vi "Boiler_Startup_Control.vi"() -> ()   [LabVIEW 2021]
doc: "This is the Main Vi that performs the boiler startup operation."
uses:
  Controls/Queue_Operation_Select.ctl
  Controls/Timer_Operation_Select.ctl
  Controls/State_and_Data.ctl
  Controls/Boiler_Status_Indicators.ctl
  Controls/Notifier_Operation_Select.ctl
  Controls/Boiler_Data.ctl
  <vilib>/Utility/file.llb/Write Delimited Spreadsheet (string).vi
panel:
  out "Boiler_Status_Indicators":T1 caption="Boiler Status Indicators"
  in  "Stop":bool
  in  "Forced_Draft_Fan":bool caption="Forced Draft Fan"
  in  "Run_Interlock":bool caption="Run Interlock"
  in  "Flame_Sensor_Value":dbl(slide) caption="Flame Sensor Value [%]" scale=0.0..100.0
  in  "Fuel_Control_Valve":dbl(knob) caption="Fuel  Control Valve Position [% Open]" scale=0.0..100.0 scale format="%.1f"
  in  "Shutdown":bool
  in  "Pilot":bool
  in  "Start_Sequence":bool caption="Start Sequence"
  in  "Boiler_Reset":bool caption="Boiler Reset"
  out "Error_Out":errorcluster
  in  "Error_In":errorcluster
  # "Boiler Controls"
  # "Boiler Simulation Controls"
  # "Closed"
  # "On"
  # "Open"
  # "Off"
  # "Boiler Start-Up steps\nStep1 : Close the interlock and hit the reset button.\nStep2 : Press the start sequence to initiate the pre-purge. \nStep3 : After the pre-purge, press the pilot button to turn on the natural gas and pilot.\nStep4 : Adjust the flame sensor to prepare the boiler.\nStep5 : Turn on the forced draft fan, then add fuel to the boiler by adjusting the fuel control valve.\nStep6 :The boiler is now started up"
  # "Seconds"
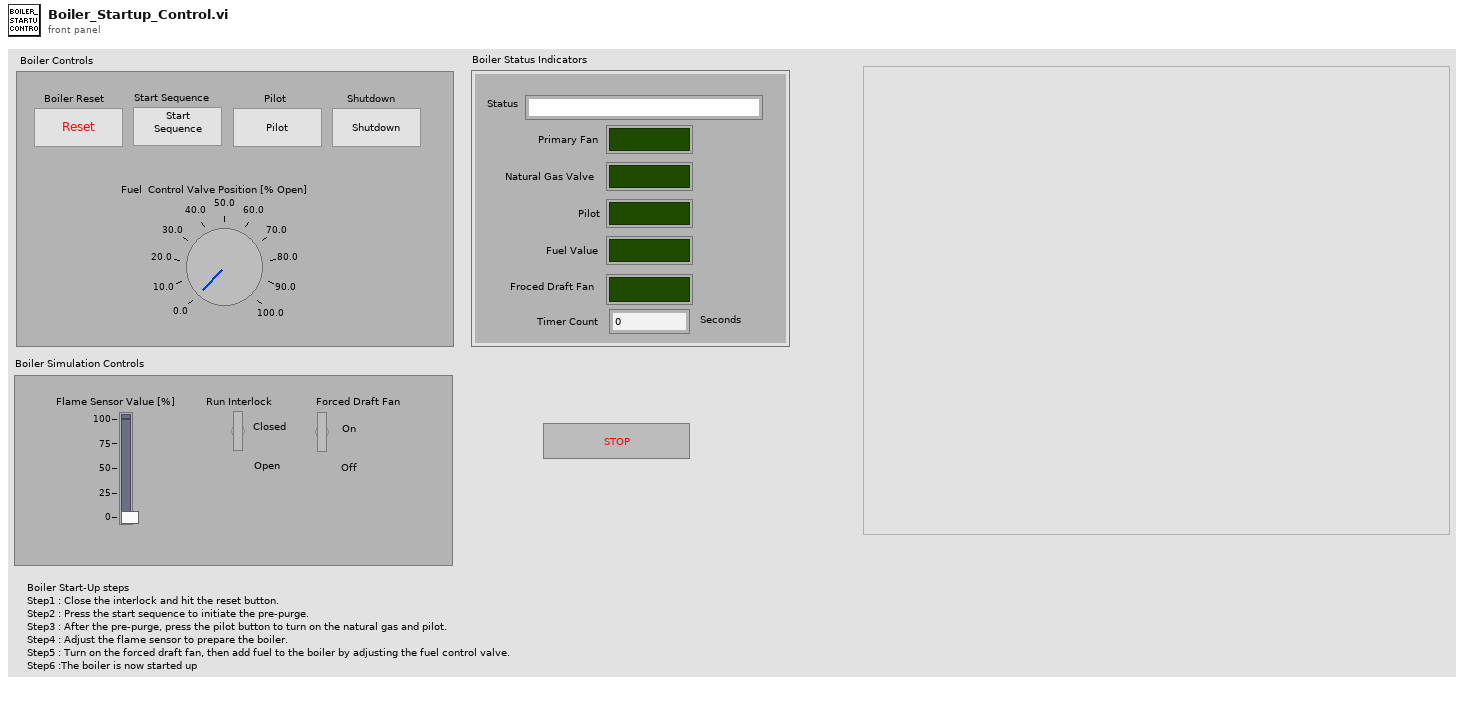
[diagram p1: front panel]
types:
  T1 = typedef "Boiler_Status_Indicators.ctl" = cluster{"Status":string, "Primary_Fan":bool, "Natural_Gas_Valve":bool, "Pilot":bool, "Fuel_Value":bool, "Froced_Draft_Fan":bool, "Timer_Count":dbl}
  T2 = typedef "Notifier_Operation_Select.ctl" = enum16{"Obtain_Notifier", "Send_Notification", "Get_Notification_Status", "Release_Notifier"}
  T3 = typedef "Queue_Operation_Select.ctl" = enum16{"Obtain_Queue", "Enqueue", "Enqueue_N", "Enqueue_at_First", "Dequeue", "Flush_Queue", "Release_Queue"}
  T4 = typedef "State_and_Data.ctl" = cluster{"State":string, "Event_Data":variant}
  T5 = typedef "Boiler_Data.ctl" = cluster{"Boiler_Status_Indicators":T1, "Start?":bool, "Pilot_On?":bool, "Blink_It?":bool, "Log_Timer_Time":bool, "ReInitialize":refnum<vi>[], "After_TimeOut_Call?":string, "Time_String":string, "Event_String":string, "Event_Data_String":string}
  T6 = typedef "Timer_Operation_Select.ctl" = enum16{"Start_Timer", "Pause_Timer", "Time_Out?", "Stop_Timer"}
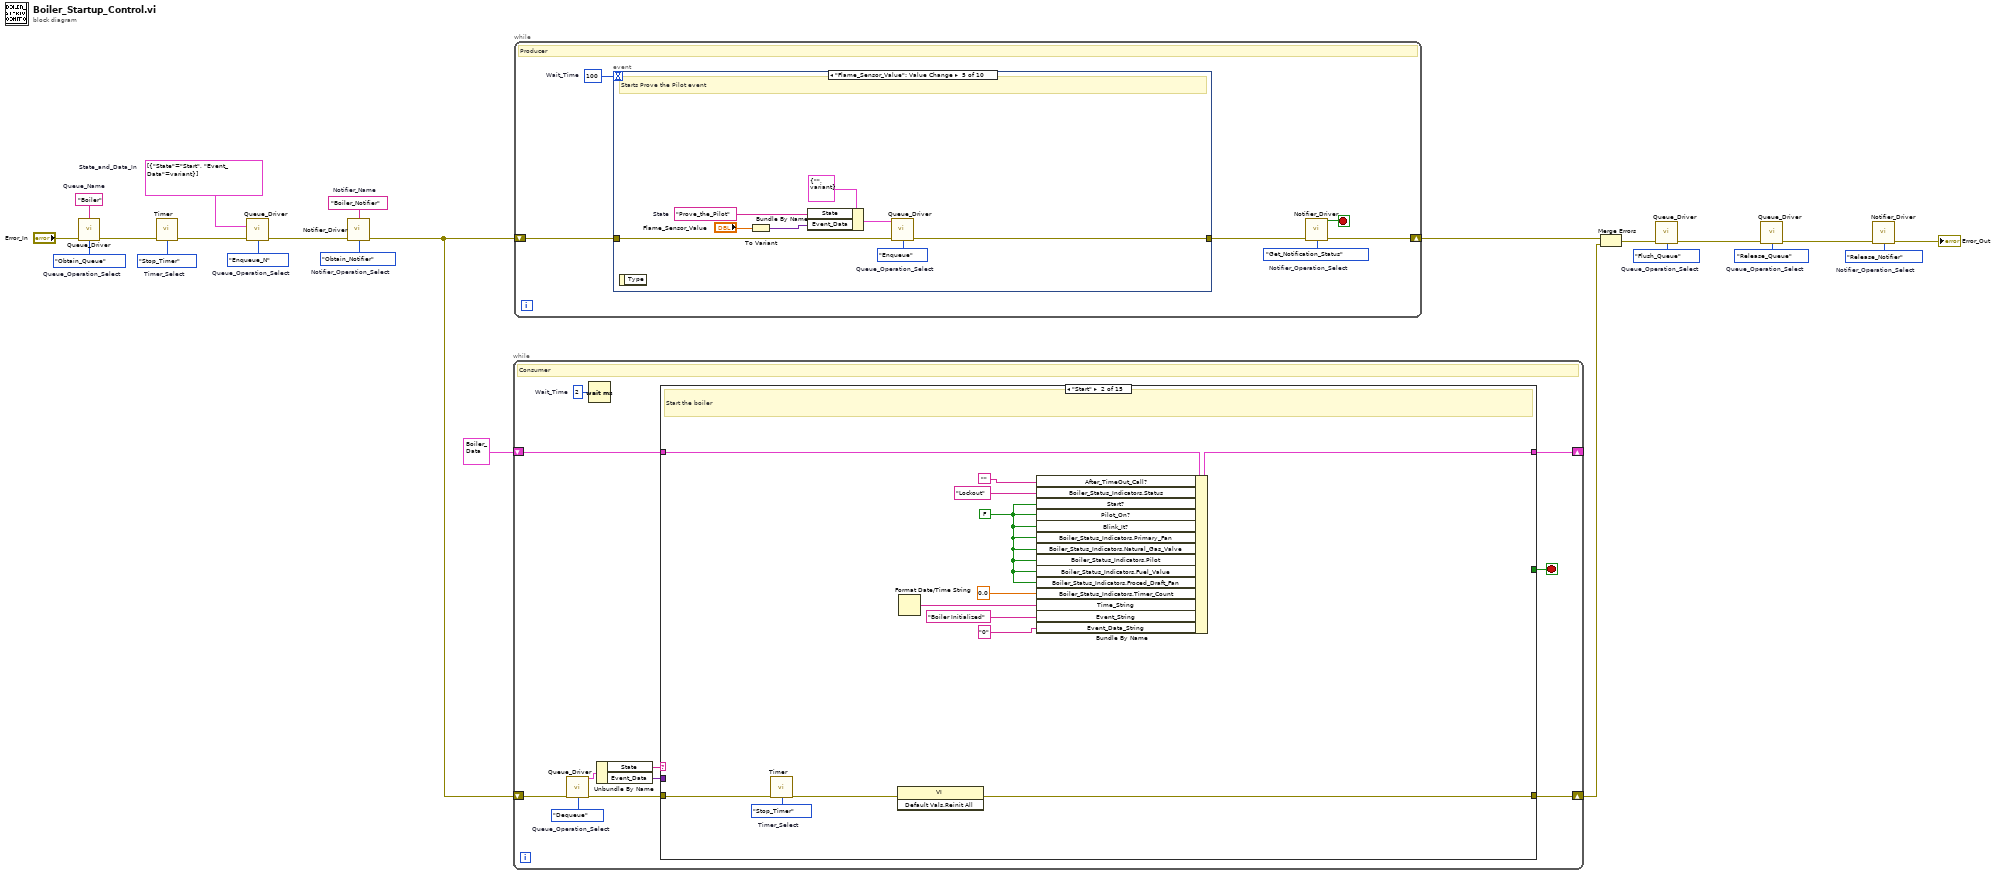
[diagram p0: block diagram]
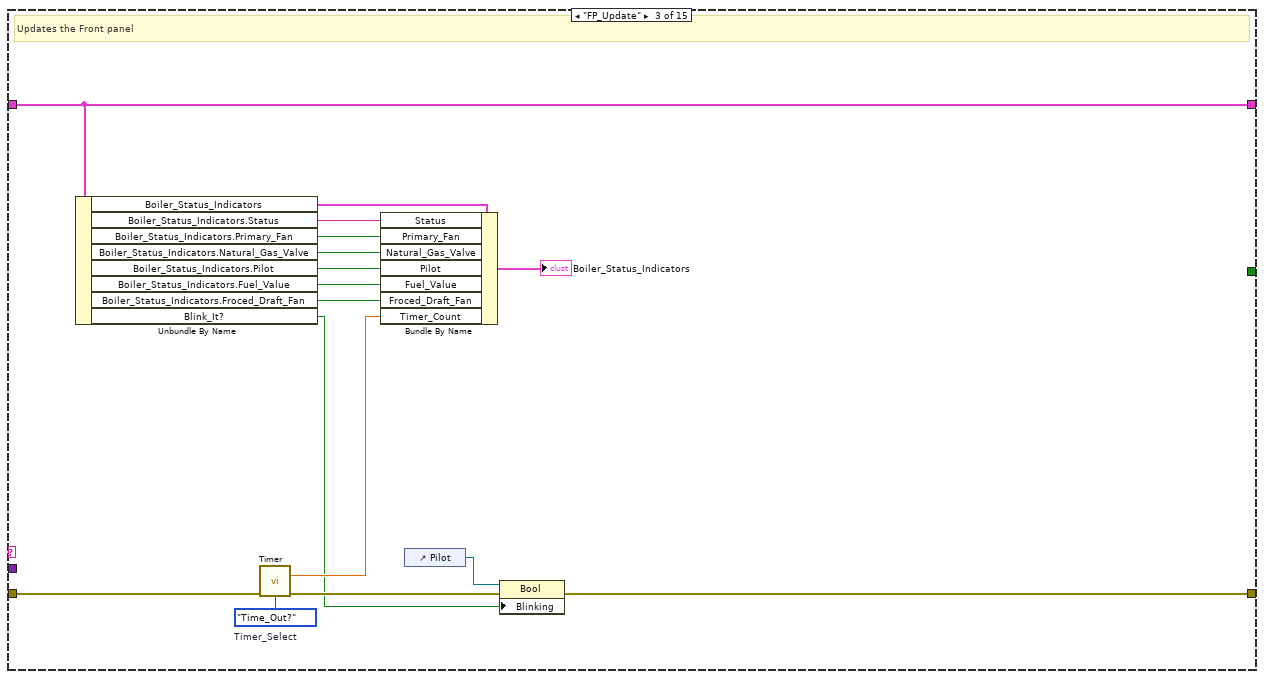
[diagram p3: hidden frame]
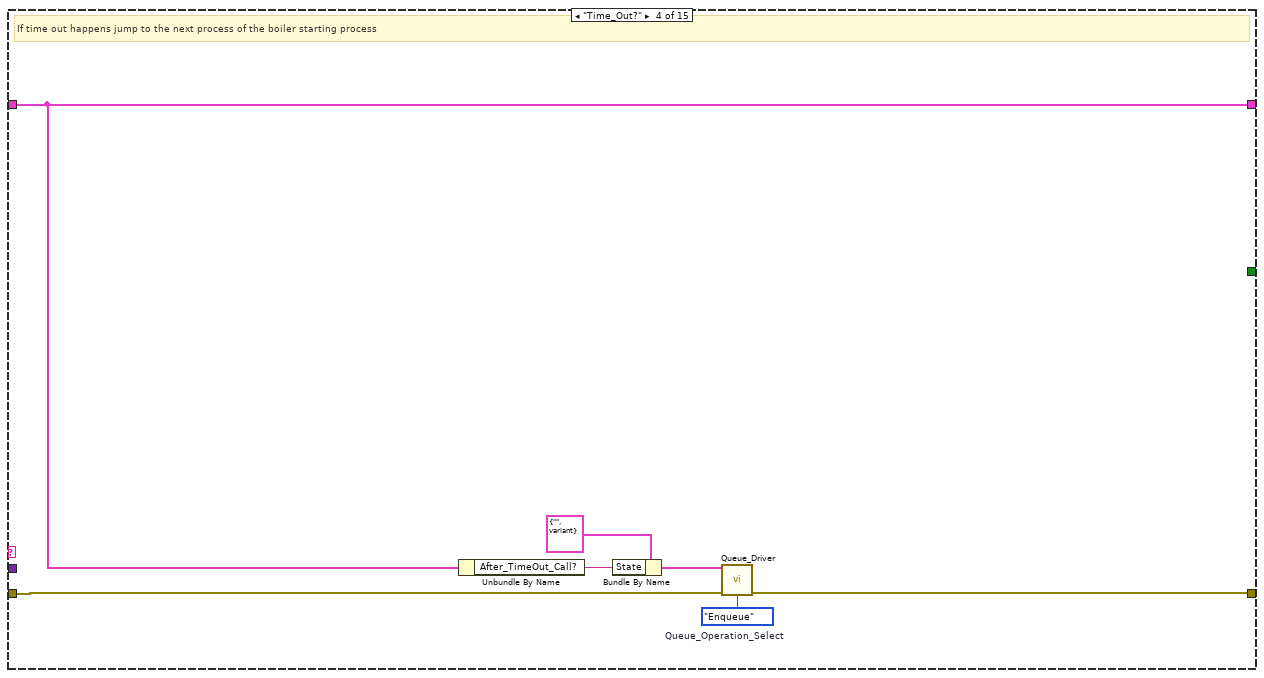
[diagram p4: hidden frame]
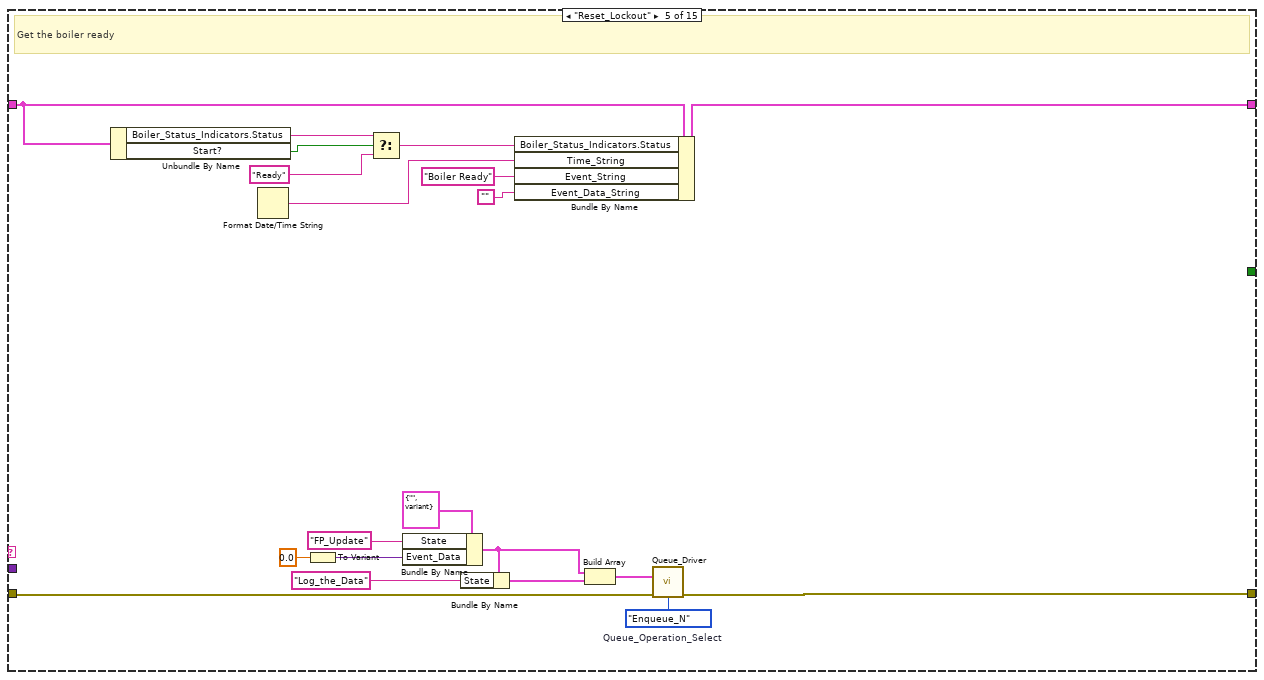
[diagram p5: hidden frame]
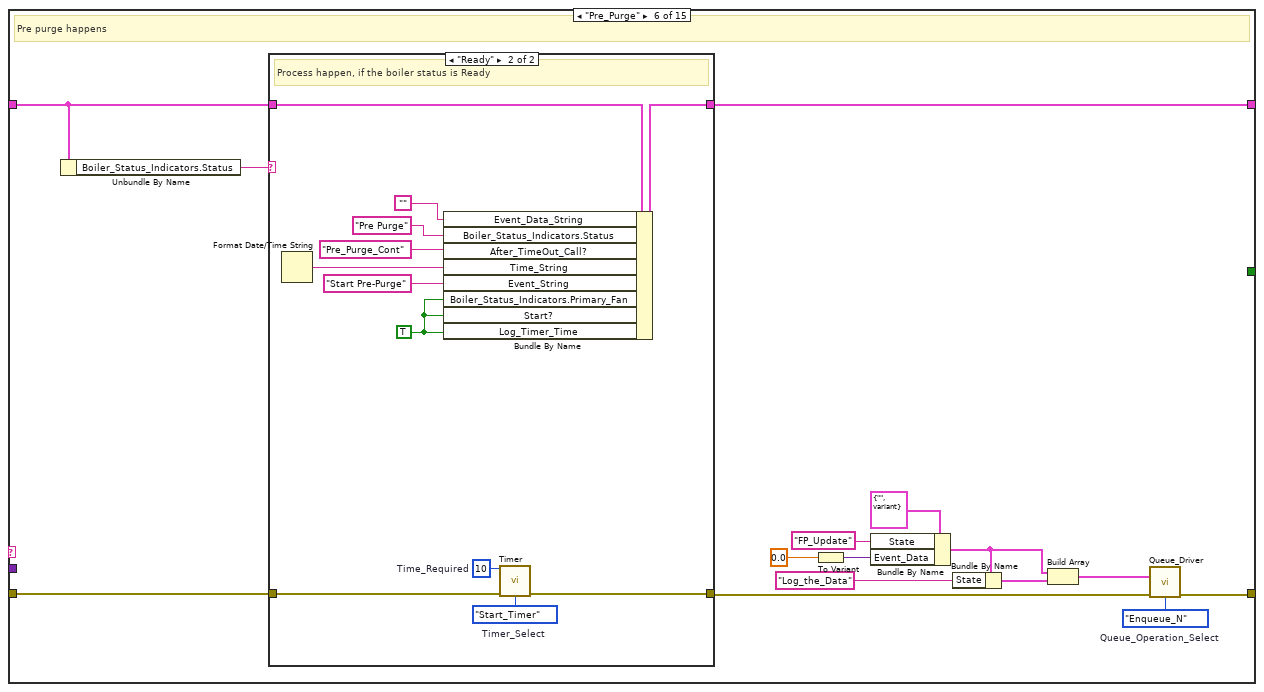
[diagram p6: hidden frame]
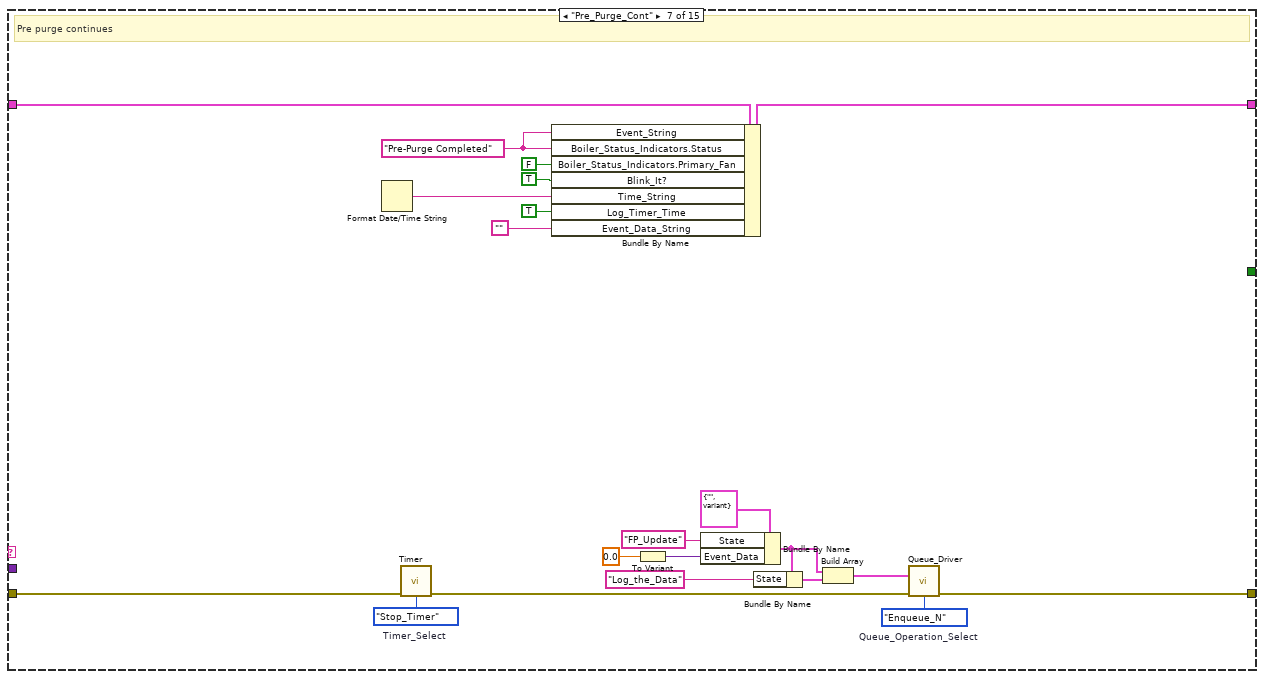
[diagram p8: hidden frame]
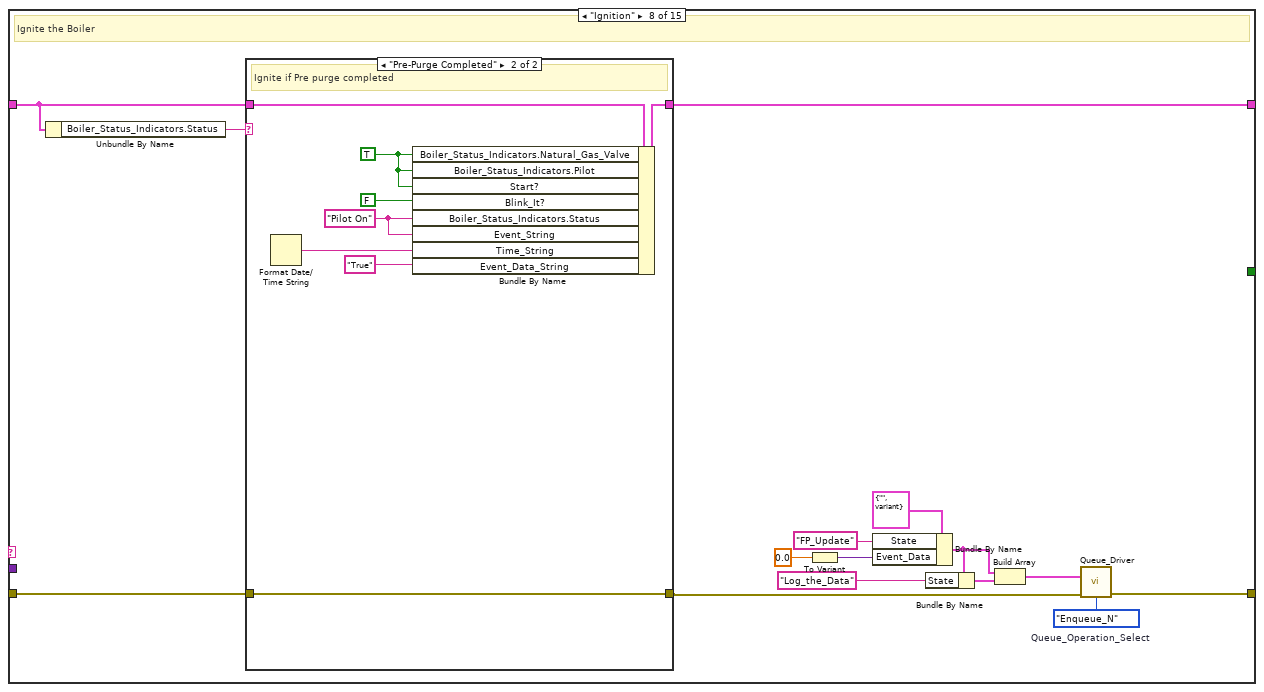
[diagram p9: hidden frame]
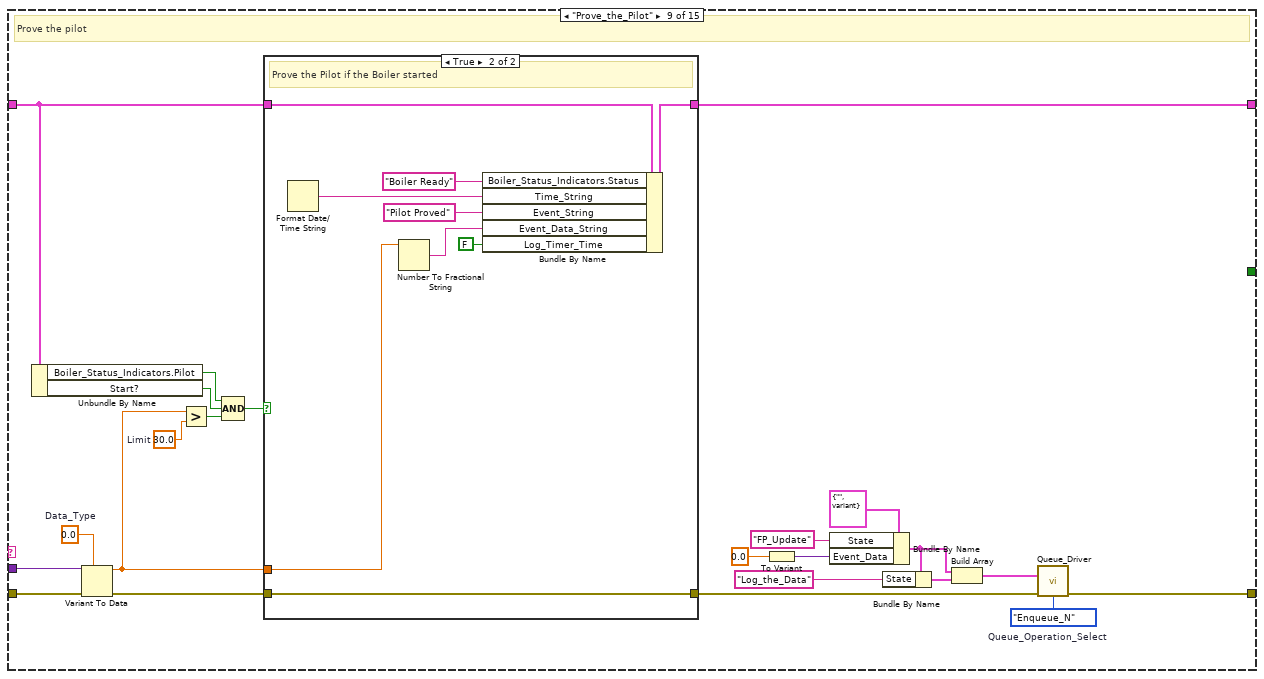
[diagram p11: hidden frame]
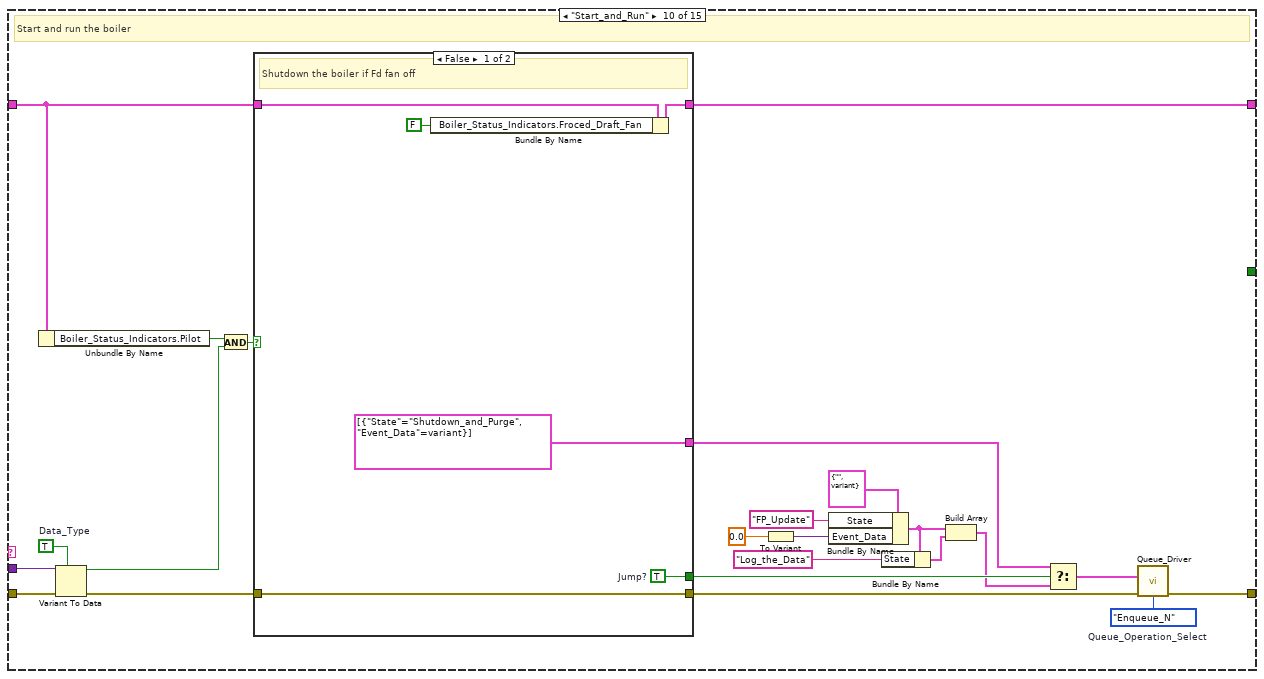
[diagram p13: hidden frame]
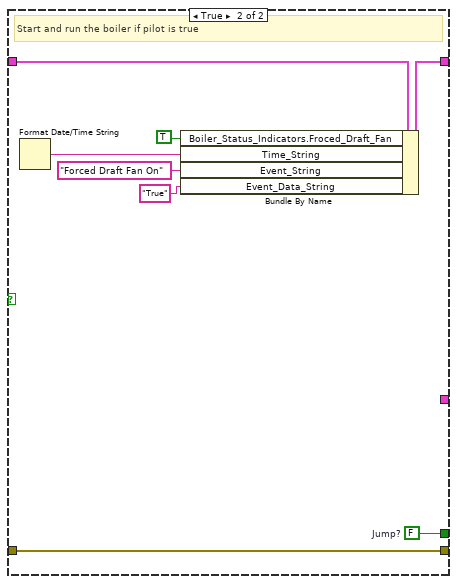
[diagram p14: hidden frame]
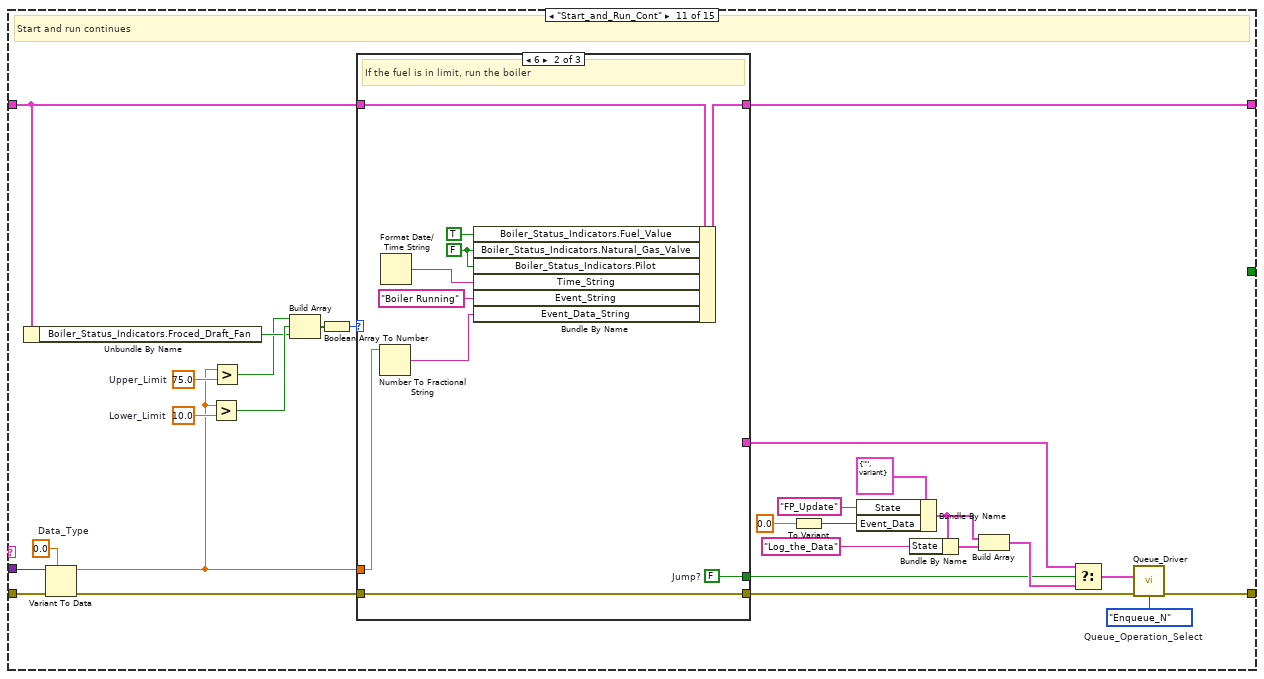
[diagram p15: hidden frame]
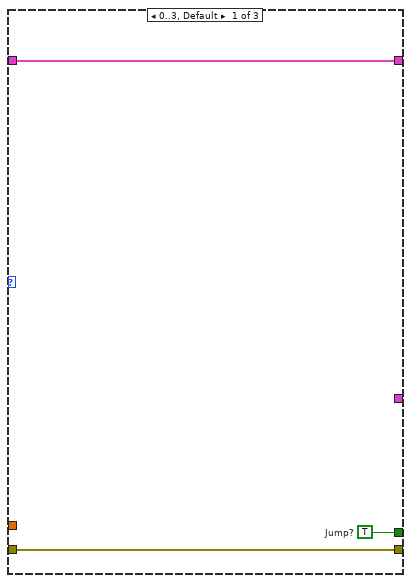
[diagram p16: hidden frame]
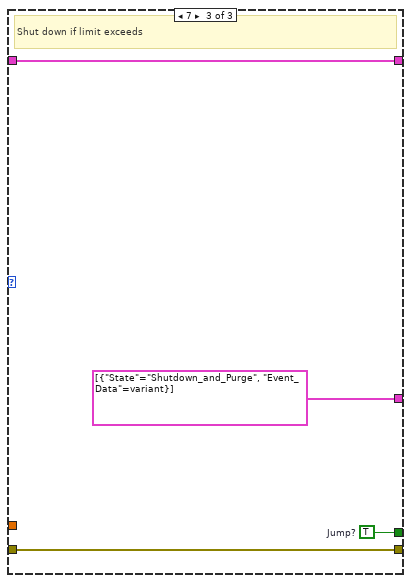
[diagram p17: hidden frame]
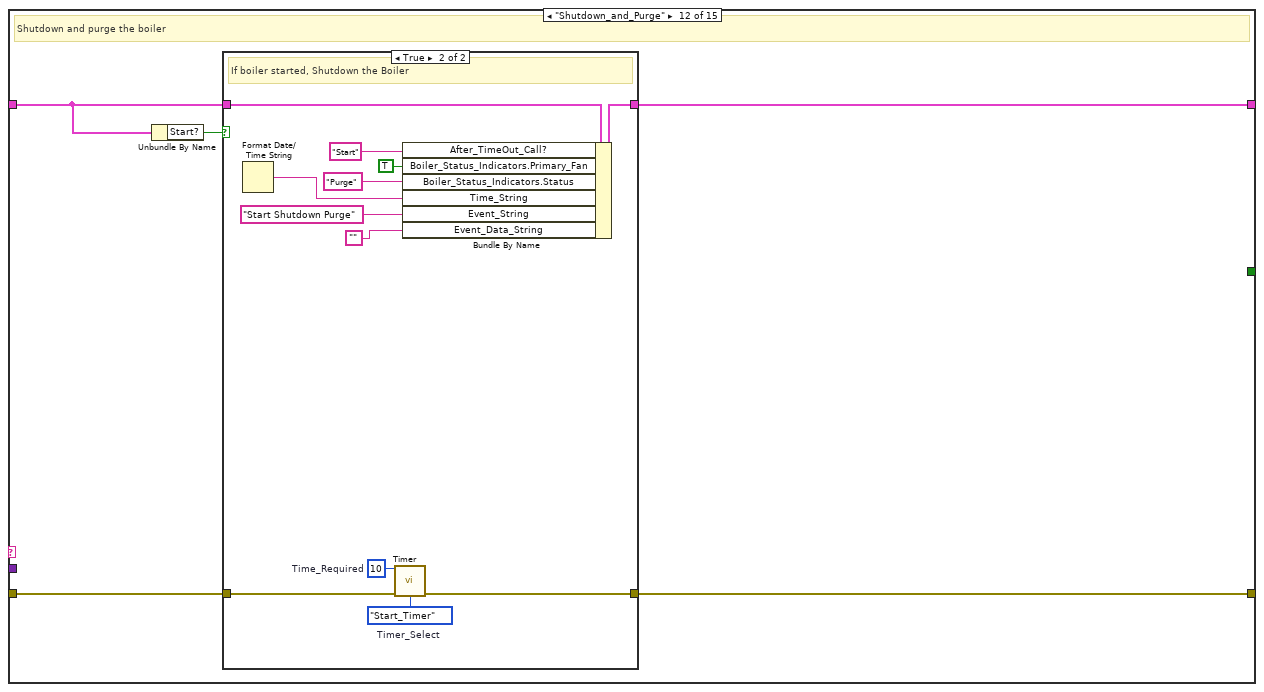
[diagram p18: hidden frame]
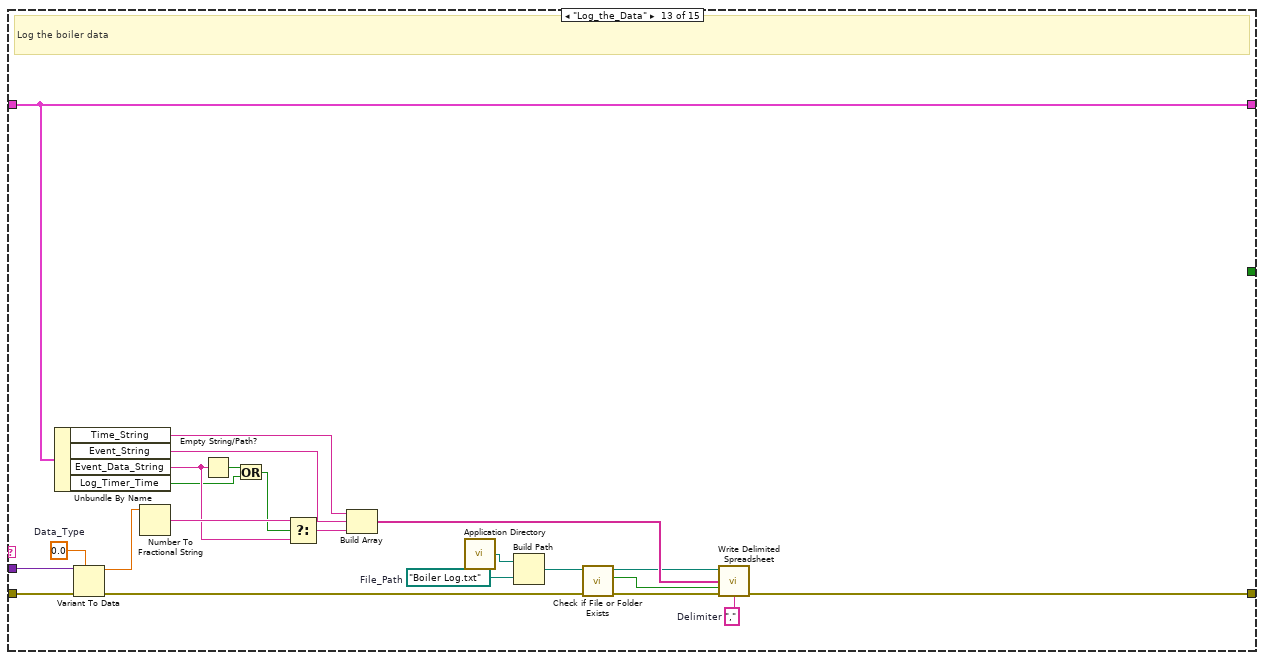
[diagram p20: hidden frame]
diagram:
  w5 = Notifier_Operation_Select."Release_Notifier"  # Notifier_Operation_Select
  w6 = Queue_Operation_Select."Release_Queue"  # Queue_Operation_Select
  w8 = Queue_Operation_Select."Flush_Queue"  # Queue_Operation_Select
  w10 = "Boiler_Notifier"  # Notifier_Name
  w11 = Notifier_Operation_Select."Obtain_Notifier"  # Notifier_Operation_Select
  w13 = T4[] [{"State"="Start", "Event_Data"=variant}]  # State_and_Data_In
  w14 = Queue_Operation_Select."Enqueue_N"  # Queue_Operation_Select
  w18 = Timer_Operation_Select."Stop_Timer"  # Timer_Select
  w19 = "Boiler"  # Queue_Name
  w20 = Queue_Operation_Select."Obtain_Queue"  # Queue_Operation_Select
  n1 = call "Queue_Driver.vi"("Queue_Name"=w19, "Error_In"="Error_In", "Queue_Operation_Select"=w20) -> ("Error_Out"=w21:errorcluster)  [unwired: 11 in, 1 out]
  n2 = call "Timer.vi"("Error_In"=w21, "Timer_Select"=w18) -> ("Error_Out"=w17:errorcluster)  [unwired: 10 in, 3 out]
  n3 = call "Queue_Driver.vi"("State_and_Data_In_N"=w13, "Error_In"=w17, "Queue_Operation_Select"=w14) -> ("Error_Out"=w15:errorcluster)  [unwired: 11 in, 1 out]
  n4 = call "Notifier_Driver.vi"("Notifier_Name"=w10, "Error_In"=w15, "Notifier_Operation_Select"=w11) -> ("Error_Out"=w12:errorcluster)  [unwired: 11 in, 1 out]
  n5 = while {
    shift-right: [w28] -> _
    shift-left: T5 {"Boiler_Status_Indicators"={"Status"="", "Primary_Fan"=FALSE, "Natural_Gas_Valve"=FALSE, "Pilot"=FALSE, "Fuel_Value"=FALSE, "Froced_Draft_Fan"=FALSE, "Timer_Count"=0.0}, "Start?"=TRUE, "Pilot_On?"=TRUE, "Blink_It?"=TRUE, "Log_Timer_Time"=FALSE, "ReInitialize"=[], "After_TimeOut_Call?"="", "Time_String"="", "Event_String"="", "Event_Data_String"=""} -> [w27]
    shift-right: [w23] -> w4
    shift-left: w12 -> [w33]
    stop <- w25 stop-if-true
    w24 = u32 2  # Wait_Time
    w31 = Queue_Operation_Select."Dequeue"  # Queue_Operation_Select
    # "Consumer"
    n6 = call "Queue_Driver.vi"("Error_In"=w33, "Queue_Operation_Select"=w31) -> ("State_and_Data_Out"=w30:T4, "Error_Out"=w32:errorcluster)  [unwired: 12 in]
    n7 = Wait (ms)(milliseconds to wait=w24) -> ()  [unwired: 1 out]
    n8 = Unbundle By Name(w30) -> ("State"=w29:string, "Event_Data"=w26:variant)
    n9 = case shown="\"Start\"" w29 {
      tunnel: w32 -> [w35 w41 w64 w68 w74 w105 w137 w154 w188 w222 w262 w286 w319 w331 w340]
      tunnel: [w35 w40 w49 w67 w73 w94 w136 w141 w167 w204 w240 w284 w323 w329 w335] -> w23
      tunnel: [w34 w48 w63 w70 w91 w106 w140 w155 w179 w221 w264 w285 w320 w330 w351] -> w28
      tunnel: w27 -> [w34 w47 w63 w70 w89 w104 w138 w153 w180 w220 w263 w283 w320 w330 w351]
      tunnel: w26 -> [_ _ _ _ _ _ _ _ w187 w217 w260 _ w318 _ _]
      tunnel: [_ _ _ _ _ _ _ _ _ _ _ _ _ w324 _] -> w25
      frame Default {
        # "Default"
      }
      frame "Start" {
        w37 = Timer_Operation_Select."Stop_Timer"  # Timer_Select
        w42 = FALSE ("Boiler_Status_Indicators.Primary_Fan")
        # "Start the boiler"
        n10 = call "Timer.vi"("Error_In"=w41, "Timer_Select"=w37) -> ("Error_Out"=w38:errorcluster)  [unwired: 10 in, 3 out]
        n11 = invoke on="Invoke Node" class="VI" method="Default Vals.Reinit All"(error in=w38) -> (error out=w40:errorcluster)  [unwired: 2 in, 2 out]
        n12 = Format Date/Time String() -> (date/time string=w36:string)  [unwired: 3 in]
        n13 = Bundle By Name(cluster=w47, "After_TimeOut_Call?"="" ("Empty String Constant"), "Boiler_Status_Indicators.Status"="Lockout", "Start?"=w42, "Pilot_On?"=w42, "Blink_It?"=w42, "Boiler_Status_Indicators.Primary_Fan"=w42, "Boiler_Status_Indicators.Natural_Gas_Valve"=w42, "Boiler_Status_Indicators.Pilot"=w42, "Boiler_Status_Indicators.Fuel_Value"=w42, "Boiler_Status_Indicators.Froced_Draft_Fan"=w42, "Boiler_Status_Indicators.Timer_Count"=0.0, "Time_String"=w36, "Event_String"="Boiler Initialized", "Event_Data_String"="0") -> (w48:T5)
      }
      frame "FP_Update" {
        w54 = Timer_Operation_Select."Time_Out?"  # Timer_Select
        # "Updates the Front panel"
        n14 = Unbundle By Name(w63) -> ("Boiler_Status_Indicators"=w62:T1, "Boiler_Status_Indicators.Status"=w61:string, "Boiler_Status_Indicators.Primary_Fan"=w60:bool, "Boiler_Status_Indicators.Natural_Gas_Valve"=w59:bool, "Boiler_Status_Indicators.Pilot"=w58:bool, "Boiler_Status_Indicators.Fuel_Value"=w57:bool, "Boiler_Status_Indicators.Froced_Draft_Fan"=w56:bool, "Blink_It?"=w51:bool)
        n15 = call "Timer.vi"("Error_In"=w64, "Timer_Select"=w54) -> ("Time"=w52:dbl, "Error_Out"=w55:errorcluster)  [unwired: 10 in, 2 out]
        n16 = Bundle By Name(cluster=w62, "Status"=w61, "Primary_Fan"=w60, "Natural_Gas_Valve"=w59, "Pilot"=w58, "Fuel_Value"=w57, "Froced_Draft_Fan"=w56, "Timer_Count"=w52) -> (→"Boiler_Status_Indicators":T1)
        n17 = control-ref of="Pilot"() -> (w50:refnum<vi>)
        n18 = property on="Property Node" class="Bool"(reference=w50, error in=w55, "Blinking"=w51) -> (error out=w49:errorcluster)  [unwired: 1 out]
      }
      frame "Time_Out?" {
        w66 = Queue_Operation_Select."Enqueue"  # Queue_Operation_Select
        # "If time out happens jump to the next process of the boiler starting process"
        n19 = Unbundle By Name(w70) -> ("After_TimeOut_Call?"=w71:string)
        n20 = Bundle By Name(cluster=T4 {"State"="", "Event_Data"=variant} ("State_and_Data_In"), "State"=w71) -> (w65:T4)
        n21 = call "Queue_Driver.vi"("State_and_Data_In"=w65, "Error_In"=w68, "Queue_Operation_Select"=w66) -> ("Error_Out"=w67:errorcluster)  [unwired: 11 in, 1 out]
      }
      frame "Reset_Lockout" {
        w82 = Queue_Operation_Select."Enqueue_N"  # Queue_Operation_Select
        # "Get the boiler ready"
        n22 = Unbundle By Name(w89) -> ("Boiler_Status_Indicators.Status"=w86:string, "Start?"=w87:bool)
        n23 = Format Date/Time String() -> (date/time string=w83:string)  [unwired: 3 in]
        n24 = To Variant(anything=0.0) -> (Variant=w77:variant)
        n25 = Select(t=w86, s=w87, f="Ready") -> (s? t:f=w88:string)
        n26 = Bundle By Name(cluster=T4 {"State"="", "Event_Data"=variant} ("State_and_Data_In"), "State"="FP_Update", "Event_Data"=w77) -> (w75:T4)
        n27 = Bundle By Name(cluster=w75, "State"="Log_the_Data") -> (w76:T4)
        n28 = Bundle By Name(cluster=w89, "Boiler_Status_Indicators.Status"=w88, "Time_String"=w83, "Event_String"="Boiler Ready", "Event_Data_String"="" ("Empty String Constant")) -> (w91:T5)
        n29 = Build Array(w75, w76) -> (w72:T4[])
        n30 = call "Queue_Driver.vi"("State_and_Data_In_N"=w72, "Error_In"=w74, "Queue_Operation_Select"=w82) -> ("Error_Out"=w73:errorcluster)  [unwired: 11 in, 1 out]
      }
      frame "Pre_Purge" {
        w96 = Queue_Operation_Select."Enqueue_N"  # Queue_Operation_Select
        # "Pre purge happens"
        n31 = Unbundle By Name(w104) -> ("Boiler_Status_Indicators.Status"=w103:string)
        n32 = case shown="\"Ready\"" w103 {
          tunnel: w104 -> [w108 w120]
          tunnel: [w108 w119] -> w106
          tunnel: w105 -> [w107 w116]
          tunnel: [w107 w115] -> w95
          frame Default {
          }
          frame "Ready" {
            w111 = TRUE ("Log_Timer_Time")
            w117 = 10  # Time_Required
            w118 = Timer_Operation_Select."Start_Timer"  # Timer_Select
            # "Process happen, if the boiler status is Ready"
            n33 = Format Date/Time String() -> (date/time string=w109:string)  [unwired: 3 in]
            n34 = Bundle By Name(cluster=w120, "Event_Data_String"="" ("Empty String Constant"), "Boiler_Status_Indicators.Status"="Pre Purge", "After_TimeOut_Call?"="Pre_Purge_Cont", "Time_String"=w109, "Event_String"="Start Pre-Purge", "Boiler_Status_Indicators.Primary_Fan"=w111, "Start?"=w111, "Log_Timer_Time"=w111) -> (w119:T5)
            n35 = call "Timer.vi"("Time_Required"=w117, "Error_In"=w116, "Timer_Select"=w118) -> ("Error_Out"=w115:errorcluster)  [unwired: 9 in, 3 out]
          }
        }
        n36 = To Variant(anything=0.0) -> (Variant=w100:variant)
        n37 = Bundle By Name(cluster=T4 {"State"="", "Event_Data"=variant} ("State_and_Data_In"), "State"="FP_Update", "Event_Data"=w100) -> (w102:T4)
        n38 = Bundle By Name(cluster=w102, "State"="Log_the_Data") -> (w101:T4)
        n39 = Build Array(w102, w101) -> (w93:T4[])
        n40 = call "Queue_Driver.vi"("State_and_Data_In_N"=w93, "Error_In"=w95, "Queue_Operation_Select"=w96) -> ("Error_Out"=w94:errorcluster)  [unwired: 11 in, 1 out]
      }
      frame "Pre_Purge_Cont" {
        w123 = Queue_Operation_Select."Enqueue_N"  # Queue_Operation_Select
        w135 = Timer_Operation_Select."Stop_Timer"  # Timer_Select
        w133 = "Pre-Purge Completed" ("Boiler_Status_Indicators.Status")
        # "Pre purge continues"
        n41 = Format Date/Time String() -> (date/time string=w130:string)  [unwired: 3 in]
        n42 = call "Timer.vi"("Error_In"=w137, "Timer_Select"=w135) -> ("Error_Out"=w136:errorcluster)  [unwired: 10 in, 3 out]
        n43 = Bundle By Name(cluster=w138, "Event_String"=w133, "Boiler_Status_Indicators.Status"=w133, "Boiler_Status_Indicators.Primary_Fan"=FALSE, "Blink_It?"=TRUE, "Time_String"=w130, "Log_Timer_Time"=TRUE, "Event_Data_String"="" ("Empty String Constant")) -> (w140:T5)
        n44 = To Variant(anything=0.0) -> (Variant=w127:variant)
        n45 = Bundle By Name(cluster=T4 {"State"="", "Event_Data"=variant} ("State_and_Data_In"), "State"="FP_Update", "Event_Data"=w127) -> (w129:T4)
        n46 = Bundle By Name(cluster=w129, "State"="Log_the_Data") -> (w128:T4)
        n47 = Build Array(w129, w128) -> (w122:T4[])
        n48 = call "Queue_Driver.vi"("State_and_Data_In_N"=w122, "Queue_Operation_Select"=w123) -> ()  [unwired: 12 in, 2 out]
      }
      frame "Ignition" {
        w145 = Queue_Operation_Select."Enqueue_N"  # Queue_Operation_Select
        # "Ignite the Boiler"
        n49 = Unbundle By Name(w153) -> ("Boiler_Status_Indicators.Status"=w152:string)
        n50 = case shown="\"Pre-Purge Completed\"" w152 {
          tunnel: w153 -> [w156 w165]
          tunnel: [w156 w164] -> w155
          tunnel: [w157 w163] -> w142
          tunnel: w154 -> [w157 w163]
          frame Default {
          }
          frame "Pre-Purge Completed" {
            w161 = "Pilot On" ("Boiler_Status_Indicators.Status")
            w162 = TRUE ("Boiler_Status_Indicators.Natural_Gas_Valve")
            # "Ignite if Pre purge completed"
            n51 = Format Date/Time String() -> (date/time string=w158:string)  [unwired: 3 in]
            n52 = Bundle By Name(cluster=w165, "Boiler_Status_Indicators.Natural_Gas_Valve"=w162, "Boiler_Status_Indicators.Pilot"=w162, "Start?"=w162, "Blink_It?"=FALSE, "Boiler_Status_Indicators.Status"=w161, "Event_String"=w161, "Time_String"=w158, "Event_Data_String"="True") -> (w164:T5)
          }
        }
        n53 = To Variant(anything=0.0) -> (Variant=w149:variant)
        n54 = Bundle By Name(cluster=T4 {"State"="", "Event_Data"=variant} ("State_and_Data_In"), "State"="FP_Update", "Event_Data"=w149) -> (w151:T4)
        n55 = Bundle By Name(cluster=w151, "State"="Log_the_Data") -> (w150:T4)
        n56 = Build Array(w151, w150) -> (w144:T4[])
        n57 = call "Queue_Driver.vi"("State_and_Data_In_N"=w144, "Error_In"=w142, "Queue_Operation_Select"=w145) -> ("Error_Out"=w141:errorcluster)  [unwired: 11 in, 1 out]
      }
      frame "Prove_the_Pilot" {
        w171 = Queue_Operation_Select."Enqueue_N"  # Queue_Operation_Select
        w184 = 30.0  # Limit
        w185 = 0.0  # Data_Type
        # "Prove the pilot"
        n58 = Unbundle By Name(w180) -> ("Boiler_Status_Indicators.Pilot"=w166:bool, "Start?"=w182:bool)
        n59 = Variant To Data(error in=w188, type=w185, Variant=w187) -> (data=w178:dbl, error out=w186:errorcluster)
        n60 = Greater?(x=w178, y=w184) -> (0:w183:bool)
        n61 = Compound Arithmetic op=AND(w166, w182, w183) -> (w181:bool)
        n62 = case shown="True" w181 {
          tunnel: [w190 w199] -> w168
          tunnel: w186 -> [w190 w199]
          tunnel: w180 -> [w189 w198]
          tunnel: [w189 w197] -> w179
          tunnel: w178 -> [_ w193]
          frame False {
          }
          frame True {
            # "Prove the Pilot if the Boiler started"
            n63 = Format Date/Time String() -> (date/time string=w191:string)  [unwired: 3 in]
            n64 = Number To Fractional String(number=w193) -> (F-format string=w194:string)  [unwired: 3 in]
            n65 = Bundle By Name(cluster=w198, "Boiler_Status_Indicators.Status"="Boiler Ready", "Time_String"=w191, "Event_String"="Pilot Proved", "Event_Data_String"=w194, "Log_Timer_Time"=FALSE) -> (w197:T5)
          }
        }
        n66 = To Variant(anything=0.0) -> (Variant=w175:variant)
        n67 = Bundle By Name(cluster=T4 {"State"="", "Event_Data"=variant} ("State_and_Data_In"), "State"="FP_Update", "Event_Data"=w175) -> (w177:T4)
        n68 = Bundle By Name(cluster=w177, "State"="Log_the_Data") -> (w176:T4)
        n69 = Build Array(w177, w176) -> (w170:T4[])
        n70 = call "Queue_Driver.vi"("State_and_Data_In_N"=w170, "Error_In"=w168, "Queue_Operation_Select"=w171) -> ("Error_Out"=w167:errorcluster)  [unwired: 11 in, 1 out]
      }
      frame "Start_and_Run" {
        w207 = Queue_Operation_Select."Enqueue_N"  # Queue_Operation_Select
        w216 = TRUE  # Data_Type
        # "Start and run the boiler"
        n71 = Unbundle By Name(w220) -> ("Boiler_Status_Indicators.Pilot"=w219:bool)
        n72 = Variant To Data(error in=w222, type=w216, Variant=w217) -> (data=w214:bool, error out=w218:errorcluster)
        n73 = And(x=w219, y=w214) -> (x .and. y?=w215:bool)
        n74 = case shown="False" w215 {
          tunnel: [w227 w236] -> w205
          tunnel: w218 -> [w227 w236]
          tunnel: [w224 w234] -> w221
          tunnel: w220 -> [w228 w235]
          tunnel: [T4[] [{"State"="Shutdown_and_Purge", "Event_Data"=variant}] _] -> w202
          tunnel: [w225 w230] -> w201
          frame False {
            w225 = TRUE  # Jump?
            # "Shutdown the boiler if Fd fan off"
            n75 = Bundle By Name(cluster=w228, "Boiler_Status_Indicators.Froced_Draft_Fan"=FALSE) -> (w224:T5)
          }
          frame True {
            w230 = FALSE  # Jump?
            # "Start and run the boiler if pilot is true"
            n76 = Format Date/Time String() -> (date/time string=w229:string)  [unwired: 3 in]
            n77 = Bundle By Name(cluster=w235, "Boiler_Status_Indicators.Froced_Draft_Fan"=TRUE, "Time_String"=w229, "Event_String"="Forced Draft Fan On", "Event_Data_String"="True") -> (w234:T5)
          }
        }
        n78 = To Variant(anything=0.0) -> (Variant=w211:variant)
        n79 = Bundle By Name(cluster=T4 {"State"="", "Event_Data"=variant} ("State_and_Data_In"), "State"="FP_Update", "Event_Data"=w211) -> (w213:T4)
        n80 = Bundle By Name(cluster=w213, "State"="Log_the_Data") -> (w212:T4)
        n81 = Build Array(w213, w212) -> (w200:T4[])
        n82 = Select(t=w202, s=w201, f=w200) -> (s? t:f=w203:T4[])
        n83 = call "Queue_Driver.vi"("State_and_Data_In_N"=w203, "Error_In"=w205, "Queue_Operation_Select"=w207) -> ("Error_Out"=w204:errorcluster)  [unwired: 11 in, 1 out]
      }
      frame "Start_and_Run_Cont" {
        w244 = Queue_Operation_Select."Enqueue_N"  # Queue_Operation_Select
        w256 = 10.0  # Lower_Limit
        w254 = 75.0  # Upper_Limit
        w259 = 0.0  # Data_Type
        # "Start and run continues"
        n84 = Unbundle By Name(w263) -> ("Boiler_Status_Indicators.Froced_Draft_Fan"=w252:bool)
        n85 = Variant To Data(error in=w262, type=w259, Variant=w260) -> (data=w253:dbl, error out=w261:errorcluster)
        n86 = Greater?(x=w253, y=w256) -> (0:w255:bool)
        n87 = Greater?(x=w253, y=w254) -> (0:w251:bool)
        n88 = Build Array(w251, w255, w252) -> (w258:bool[])
        n89 = Boolean Array To Number(Boolean array=w258) -> (number=w257:u32)
        n90 = case shown="6" w257 {
          tunnel: w263 -> [w266 w277 w281]
          tunnel: [w266 w276 w281] -> w264
          tunnel: [w267 w275 w280] -> w241
          tunnel: w261 -> [w267 w275 w280]
          tunnel: [_ _ T4[] [{"State"="Shutdown_and_Purge", "Event_Data"=variant}]] -> w237
          tunnel: w253 -> [_ w270 _]
          tunnel: [w265 w269 w278] -> w238
          frame 0..3, Default {
            w265 = TRUE  # Jump?
          }
          frame 6 {
            w269 = FALSE  # Jump?
            w273 = FALSE ("Boiler_Status_Indicators.Natural_Gas_Valve")
            # "If the fuel is in limit, run the boiler"
            n91 = Number To Fractional String(number=w270) -> (F-format string=w271:string)  [unwired: 3 in]
            n92 = Format Date/Time String() -> (date/time string=w268:string)  [unwired: 3 in]
            n93 = Bundle By Name(cluster=w277, "Boiler_Status_Indicators.Fuel_Value"=TRUE, "Boiler_Status_Indicators.Natural_Gas_Valve"=w273, "Boiler_Status_Indicators.Pilot"=w273, "Time_String"=w268, "Event_String"="Boiler Running", "Event_Data_String"=w271) -> (w276:T5)
          }
          frame 7 {
            w278 = TRUE  # Jump?
            # "Shut down if limit exceeds"
          }
        }
        n94 = To Variant(anything=0.0) -> (Variant=w248:variant)
        n95 = Bundle By Name(cluster=T4 {"State"="", "Event_Data"=variant} ("State_and_Data_In"), "State"="FP_Update", "Event_Data"=w248) -> (w250:T4)
        n96 = Bundle By Name(cluster=w250, "State"="Log_the_Data") -> (w249:T4)
        n97 = Build Array(w250, w249) -> (w243:T4[])
        n98 = Select(t=w237, s=w238, f=w243) -> (s? t:f=w239:T4[])
        n99 = call "Queue_Driver.vi"("State_and_Data_In_N"=w239, "Error_In"=w241, "Queue_Operation_Select"=w244) -> ("Error_Out"=w240:errorcluster)  [unwired: 11 in, 1 out]
      }
      frame "Shutdown_and_Purge" {
        # "Shutdown and purge the boiler"
        n100 = Unbundle By Name(w283) -> ("Start?"=w282:bool)
        n101 = case shown="True" w282 {
          tunnel: w286 -> [w287 w300]
          tunnel: w283 -> [w288 w299]
          tunnel: [w288 w298] -> w285
          tunnel: [w287 w297] -> w284
          frame False {
          }
          frame True {
            w295 = 10  # Time_Required
            w296 = Timer_Operation_Select."Start_Timer"  # Timer_Select
            # "If boiler started, Shutdown the Boiler"
            n102 = Format Date/Time String() -> (date/time string=w289:string)  [unwired: 3 in]
            n103 = call "Timer.vi"("Time_Required"=w295, "Error_In"=w300, "Timer_Select"=w296) -> ("Error_Out"=w297:errorcluster)  [unwired: 9 in, 3 out]
            n104 = Bundle By Name(cluster=w299, "After_TimeOut_Call?"="Start", "Boiler_Status_Indicators.Primary_Fan"=TRUE, "Boiler_Status_Indicators.Status"="Purge", "Time_String"=w289, "Event_String"="Start Shutdown Purge", "Event_Data_String"="" ("Empty String Constant")) -> (w298:T5)
          }
        }
      }
      frame "Log_the_Data" {
        w317 = 0.0  # Data_Type
        w321 = path "Boiler Log.txt"  # File_Path
        w322 = ","  # Delimiter
        # "Log the boiler data"
        n105 = Unbundle By Name(w320) -> ("Time_String"=w315:string, "Event_String"=w314:string, "Event_Data_String"=w310:string, "Log_Timer_Time"=w308:bool)
        n106 = Variant To Data(error in=w319, type=w317, Variant=w318) -> (data=w313:dbl, error out=w301:errorcluster)
        n107 = Number To Fractional String(number=w313) -> (F-format string=w312:string)  [unwired: 3 in]
        n108 = Empty String/Path?(string/path=w310) -> (empty?=w309:bool)
        n109 = Or(x=w309, y=w308) -> (x .or. y?=w307:bool)
        n110 = Select(t=w312, s=w307, f=w310) -> (s? t:f=w311:string)
        n111 = Build Array(w315, w314, w311) -> (w316:string[])
        n112 = call <vilib>:"Application Directory.vi"() -> ("Application Directory"=w302:path)
        n113 = Build Path(base path=w302, name or relative path=w321) -> (appended path=w305:path)
        n114 = call <vilib>:"Check if File or Folder Exists.vi"("error in (no error)"=w301, "path"=w305) -> ("error out"=w306:errorcluster, "file or folder exists?"=w303:bool, "dup path"=w304:path)  [unwired: 7 in]
        n115 = call-poly <vilib>:"Write Delimited Spreadsheet.vi"("file path (dialog if empty)"=w304, "1D data"=w316, "append to file? (new file:F)"=w303, "error in (no error)"=w306, "delimiter (\\t)"=w322) -> ("error out"=w323:errorcluster)  [unwired: 9 in, 1 out]
      }
      frame "Exit" {
        w327 = "No"  # Back
        w326 = "Yes"  # Stop_Execution
        w328 = Notifier_Operation_Select."Send_Notification"  # Notifier_Operation_Select
        # "Close the Application"
        n116 = disable-structure "Conditional Disable Structure" shown="RUN_TIME_ENGINE==True" {
          disable-tunnel: [w332 "Do you want to Exit" ("Message")] -> w325
          frame condition #0 (active) {
            w332 = "Do you want to stop the execution"  # Message
            # "Developer mode"
          }
          frame condition #1 {
            # "Run time engine mode"
          }
        }
        n117 = Two Button Dialog(message=w325, 1:w327, 2:w326) -> (T button?=w324:bool)
        n118 = call "Notifier_Driver.vi"("Notification"=w324, "Error_In"=w331, "Notifier_Operation_Select"=w328) -> ("Error_Out"=w329:errorcluster)  [unwired: 11 in, 1 out]
      }
      frame "Error" {
        w337 = Queue_Operation_Select."Enqueue_N"  # Queue_Operation_Select
        w345 = "%d%s%s"  # Format_String
        w346 = "Application Error"  # Initial_String
        w347 = "Stop"  # T_Button
        w348 = "Continue"  # F_Button
        w350 = T4[] [{"State"="Exit", "Event_Data"=variant}]  # State_and_Data_In
        # "Handles the error"
        n119 = call <vilib>:"Clear Errors.vi"("error in (no error)"=w340) -> ("error out"=w343:errorcluster)  [unwired: 5 in, 1 out]
        n120 = Unbundle By Name(w340) -> ("code"=w342:i32, "source"=w341:string)
        n121 = Format Into String(format string=w345, initial string=w346, error in=w343, w342, "\n" ("Line Feed Constant"), w341) -> (resulting string=w349:string, error out=w336:errorcluster)
        n122 = Two Button Dialog(message=w349, 1:w348, 2:w347) -> (T button?=w339:bool)
        n123 = Select(t=w350, s=w339, f=T4[] []) -> (s? t:f=w334:T4[])
        n124 = call "Queue_Driver.vi"("State_and_Data_In_N"=w334, "Error_In"=w336, "Queue_Operation_Select"=w337) -> ("Error_Out"=w335:errorcluster)  [unwired: 11 in, 1 out]
      }
    }
  }
  n125 = while {
    shift-right: [w352] -> w3
    shift-left: w12 -> [w357]
    stop <- w354 stop-if-true
    w355 = Notifier_Operation_Select."Get_Notification_Status"  # Notifier_Operation_Select
    w356 = 100  # Wait_Time
    # "Producer"
    n126 = event shown="[4] \"Flame_Sensor_Value\": Value Change" {
      selector: _ -> [_ _ _ _ _ _ _ _ _ _]
      dyn-events: _ -> [_ _ _ _ _ _ _ _ _ _]
      timeout: w356 -> [_ _ _ _ _ _ _ _ _ _]
      tunnel: w357 -> [w369 w389 w399 w403 w411 w419 w424 w431 w435 w440]
      tunnel: [w358 w382 w396 w400 w405 w413 w421 w428 w432 w436] -> w353
      event Timeout {
        w366 = Queue_Operation_Select."Enqueue_N"  # Queue_Operation_Select
        w367 = Timer_Operation_Select."Time_Out?"  # Timer_Select
        # "Check for timer"
        n127 = event-data() -> ()  [unwired: 1 in, 1 out]
        n128 = call "Timer.vi"("Error_In"=w369, "Timer_Select"=w367) -> ("Time_Out?"=w364:bool, "Time"=w363:dbl, "Start?"=w360:bool, "Error_Out"=w368:errorcluster)  [unwired: 10 in]
        n129 = Build Array(w364, w360) -> (w361:bool[])
        n130 = Boolean Array To Number(Boolean array=w361) -> (number=w359:u32)
        n131 = case shown="2" w359 {
          tunnel: w368 -> [w370 w379 w381]
          tunnel: [w370 w379 w381] -> w365
          tunnel: [_ w376 w380] -> w362
          tunnel: w363 -> [_ w378 _]
          frame 0, Default {
          }
          frame 2 {
            w371 = T4 {"State"="", "Event_Data"=variant} ("State_and_Data_In")
            # "If the timer started, update FP and log"
            n132 = To Variant(anything=w378) -> (Variant=w374:variant)
            n133 = Bundle By Name(cluster=w371, "State"="FP_Update", "Event_Data"=w374) -> (w377:T4)
            n134 = Bundle By Name(cluster=w371, "State"="Log_the_Data", "Event_Data"=w374) -> (w372:T4)
            n135 = Build Array(w377, w372) -> (w376:T4[])
          }
          frame 3 {
            w380 = T4[] [{"State"="Time_Out?", "Event_Data"=variant}]  # States_and_Data
            # "If Timer timeout, jump to timeout"
          }
        }
        n136 = call "Queue_Driver.vi"("State_and_Data_In_N"=w362, "Error_In"=w365, "Queue_Operation_Select"=w366) -> ("Error_Out"=w358:errorcluster)  [unwired: 11 in, 1 out]
      }
      event "Run_Interlock", "Boiler_Reset": Value Change {
        # "Starts the Reset and lockout, if run interlocked"
        n137 = event-data() -> ()  [unwired: 1 in, 1 out]
        n138 = Build Array("Boiler_Reset", "Run_Interlock") -> (w387:bool[])
        n139 = Boolean Array To Number(Boolean array=w387) -> (number=w386:u32)
        n140 = case shown="3" w386 {
          tunnel: w389 -> [w391 w393 w395]
          tunnel: [w391 w393 w395] -> w388
          tunnel: [_ w392 w394] -> w384
          frame Default {
          }
          frame 0 {
            w392 = T4 {"State"="Shutdown_and_Purge", "Event_Data"=variant}  # State_and_Data_In
            # "Jump to Shutdown_and_Purge if run interlock opened"
          }
          frame 3 {
            w394 = T4 {"State"="Reset_Lockout", "Event_Data"=variant}  # State_and_Data_In
            # "Jump to Reset lockout, if run interlock closed"
          }
        }
        n141 = call "Queue_Driver.vi"("State_and_Data_In"=w384, "Error_In"=w388, "Queue_Operation_Select"=Queue_Operation_Select."Enqueue") -> ("Error_Out"=w382:errorcluster)  [unwired: 11 in, 1 out]
      }
      event "Start_Sequence": Value Change {
        w398 = Queue_Operation_Select."Enqueue"  # Queue_Operation_Select
        # "Starts the Pre Purge event"
        n142 = event-data() -> ()  [unwired: 1 in, 1 out]
        n143 = call "Queue_Driver.vi"("State_and_Data_In"=T4 {"State"="Pre_Purge", "Event_Data"=variant}, "Error_In"=w399, "Queue_Operation_Select"=w398) -> ("Error_Out"=w396:errorcluster)  [unwired: 11 in, 1 out]
      }
      event "Pilot": Value Change {
        w401 = T4 {"State"="Ignition", "Event_Data"=variant}  # State_and_Data_In
        w402 = Queue_Operation_Select."Enqueue"  # Queue_Operation_Select
        # "Starts the ignition event"
        n144 = event-data() -> ()  [unwired: 1 in, 1 out]
        n145 = call "Queue_Driver.vi"("State_and_Data_In"=w401, "Error_In"=w403, "Queue_Operation_Select"=w402) -> ("Error_Out"=w400:errorcluster)  [unwired: 11 in, 1 out]
      }
      event "Flame_Sensor_Value": Value Change {
        w408 = "Prove_the_Pilot"  # State
        w410 = Queue_Operation_Select."Enqueue"  # Queue_Operation_Select
        # "Starts Prove the Pilot event"
        n146 = event-data() -> ()  [unwired: 1 in, 1 out]
        n147 = To Variant(anything="Flame_Sensor_Value") -> (Variant=w406:variant)
        n148 = Bundle By Name(cluster=T4 {"State"="", "Event_Data"=variant} ("State_and_Data_In"), "State"=w408, "Event_Data"=w406) -> (w409:T4)
        n149 = call "Queue_Driver.vi"("State_and_Data_In"=w409, "Error_In"=w411, "Queue_Operation_Select"=w410) -> ("Error_Out"=w405:errorcluster)  [unwired: 11 in, 1 out]
      }
      event "Forced_Draft_Fan": Value Change {
        w418 = Queue_Operation_Select."Enqueue"  # Queue_Operation_Select
        # "Starts the Start and run event"
        n150 = event-data() -> ()  [unwired: 1 in, 1 out]
        n151 = To Variant(anything="Forced_Draft_Fan") -> (Variant=w414:variant)
        n152 = Bundle By Name(cluster=T4 {"State"="", "Event_Data"=variant} ("State_and_Data_In"), "State"="Start_and_Run", "Event_Data"=w414) -> (w417:T4)
        n153 = call "Queue_Driver.vi"("State_and_Data_In"=w417, "Error_In"=w419, "Queue_Operation_Select"=w418) -> ("Error_Out"=w413:errorcluster)  [unwired: 11 in, 1 out]
      }
      event "Fuel_Control_Valve": Value Change {
        w425 = "Start_and_Run_Cont"  # State
        w427 = Queue_Operation_Select."Enqueue"  # Queue_Operation_Select
        # "Starts the Start and run event Cont"
        n154 = event-data() -> ()  [unwired: 1 in, 1 out]
        n155 = To Variant(anything="Fuel_Control_Valve") -> (Variant=w422:variant)
        n156 = Bundle By Name(cluster=T4 {"State"="", "Event_Data"=variant} ("State_and_Data_In"), "State"=w425, "Event_Data"=w422) -> (w426:T4)
        n157 = call "Queue_Driver.vi"("State_and_Data_In"=w426, "Error_In"=w424, "Queue_Operation_Select"=w427) -> ("Error_Out"=w421:errorcluster)  [unwired: 11 in, 1 out]
      }
      event "Shutdown": Value Change {
        w429 = T4 {"State"="Shutdown_and_Purge", "Event_Data"=variant}  # State_and_Data_In
        w430 = Queue_Operation_Select."Enqueue"  # Queue_Operation_Select
        # "Shutdown the system"
        n158 = event-data() -> ()  [unwired: 1 in, 1 out]
        n159 = call "Queue_Driver.vi"("State_and_Data_In"=w429, "Error_In"=w431, "Queue_Operation_Select"=w430) -> ("Error_Out"=w428:errorcluster)  [unwired: 11 in, 1 out]
      }
      event "Stop": Value Change {
        w433 = T4 {"State"="Exit", "Event_Data"=variant}  # State_and_Data_In
        w434 = Queue_Operation_Select."Enqueue"  # Queue_Operation_Select
        # "If stop pressed, jump to Exit"
        n160 = event-data() -> ()  [unwired: 1 in, 1 out]
        n161 = call "Queue_Driver.vi"("State_and_Data_In"=w433, "Error_In"=w435, "Queue_Operation_Select"=w434) -> ("Error_Out"=w432:errorcluster)  [unwired: 11 in, 1 out]
      }
      event Panel Close? {
        w438 = T4 {"State"="Exit", "Event_Data"=variant}  # State_and_Data_In
        w439 = Queue_Operation_Select."Enqueue"  # Queue_Operation_Select
        # "If panel closed, Jump to Exit"
        n162 = event-data() -> ()  [unwired: 1 in, 1 out]
        n163 = call "Queue_Driver.vi"("State_and_Data_In"=w438, "Error_In"=w440, "Queue_Operation_Select"=w439) -> ("Error_Out"=w436:errorcluster)  [unwired: 11 in, 1 out]
        n164 = event-data ("Event Filter Node")("Discard?"=TRUE) -> ()  [unwired: 1 in, 1 out]
      }
    }
    n165 = call "Notifier_Driver.vi"("Error_In"=w353, "Notifier_Operation_Select"=w355) -> ("Latest_Notification"=w354:bool, "Error_Out"=w352:errorcluster)  [unwired: 12 in]
  }
  n166 = Merge Errors(w3, w4) -> (w2:errorcluster)
  n167 = call "Queue_Driver.vi"("Error_In"=w2, "Queue_Operation_Select"=w8) -> ("Error_Out"=w9:errorcluster)  [unwired: 12 in, 1 out]
  n168 = call "Queue_Driver.vi"("Error_In"=w9, "Queue_Operation_Select"=w6) -> ("Error_Out"=w7:errorcluster)  [unwired: 12 in, 1 out]
  n169 = call "Notifier_Driver.vi"("Error_In"=w7, "Notifier_Operation_Select"=w5) -> ("Error_Out"=→"Error_Out":errorcluster)  [unwired: 12 in, 1 out]
